vi "反控启动.vi"(10 "启动参数":T1(ring)=enum."CODCr", 11 "启动类型":T2(ring)) -> ()   [LabVIEW 2016]
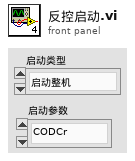
[diagram p1: front panel]
types:
  T1 = enum16{"未选择", "CODMn", "氨氮", "总磷", "总氮", "CODCr"}
  T2 = enum16{"启动整机", "停止整机", "标样核查", "加标回收", "平行样测试", "零点核查", "跨度核查", "校零", "校标"}
  T3 = cluster{"测量模式":enum16{"水样测量", "标样核查", "零点核查", "跨度核查", "空白测试", "加标回收", "平行样", "校零", "校标"}}
  T4 = cluster{"站号":u16, "量程切换":enum32{"H", "L", "AUTO"}, "控制命令":enum16{"启动测量", "标样核查", "零点核查", "跨度核查", "空白测试", "平行样测试", "加标回收", "空白校准", "标样校准", "初始化（清洗）", "停止测试", "仪器重启", "校时", "模式设置", "测量间隔设置"}, "模式设置":enum16{"待机", "连续模式", "周期模式", "定点模式", "受控模式", "手动模式"}, "测量间隔":u16}
  T5 = cluster{"status":bool, "代码":u16, "source":string}
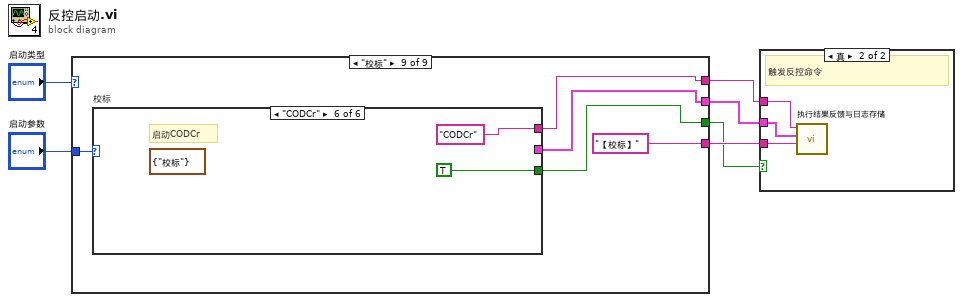
[diagram p0: block diagram]
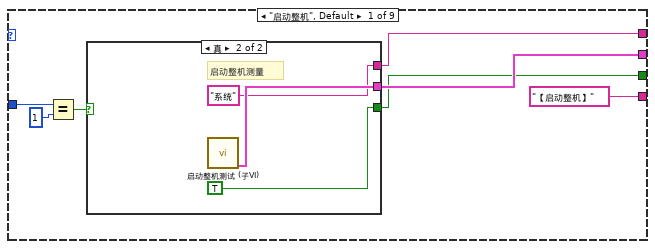
[diagram p3: hidden frame]
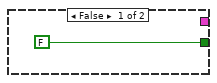
[diagram p4: hidden frame]
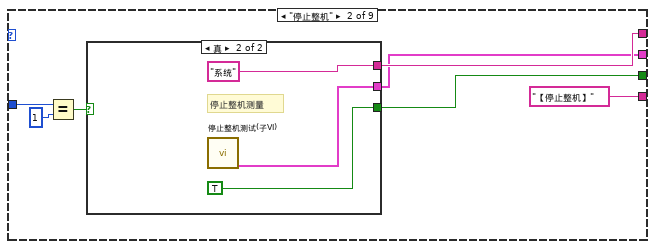
[diagram p5: hidden frame]
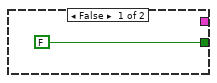
[diagram p6: hidden frame]
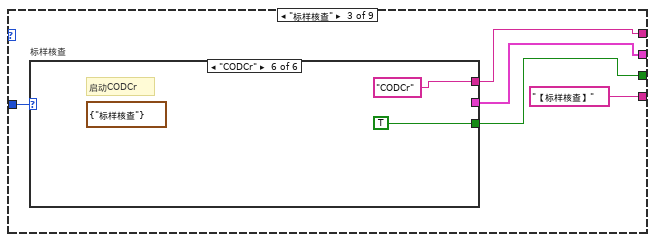
[diagram p7: hidden frame]
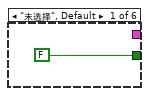
[diagram p8: hidden frame]
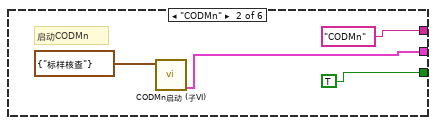
[diagram p9: hidden frame]
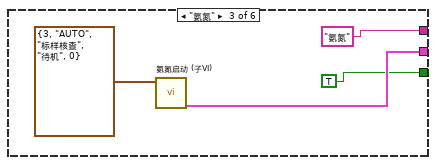
[diagram p10: hidden frame]
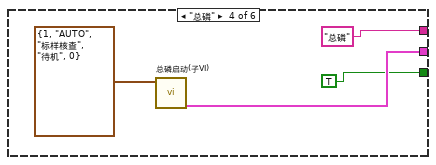
[diagram p11: hidden frame]
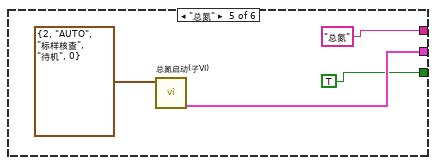
[diagram p12: hidden frame]
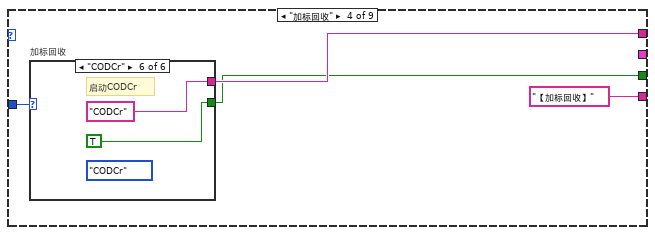
[diagram p13: hidden frame]
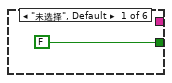
[diagram p14: hidden frame]
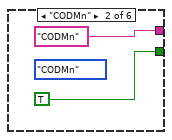
[diagram p15: hidden frame]
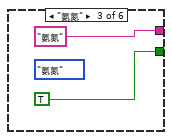
[diagram p16: hidden frame]
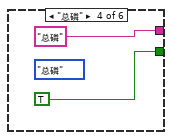
[diagram p17: hidden frame]
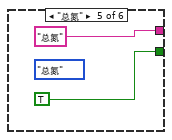
[diagram p18: hidden frame]
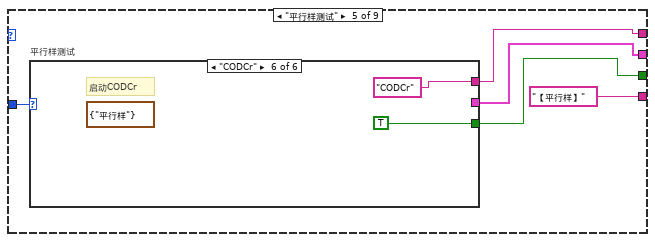
[diagram p19: hidden frame]
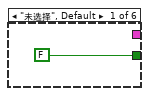
[diagram p20: hidden frame]
diagram:
  n1 = case shown="\"校标\"" "启动类型" {
    tunnel: "启动参数" -> [w13 w23 w33 w55 w72 w96 w120 w143 w168]
    tunnel: ["【启动整机】" ("日志信息") "【停止整机】" ("日志信息") "【标样核查】" ("日志信息") "【加标回收】" ("日志信息") "【平行样】" ("日志信息") "【零点核查】" ("日志信息") "【跨度核查】" ("日志信息") "【校零】" ("日志信息") "【校标】" ("日志信息")] -> w4
    tunnel: [w7 w19 w31 w53 w70 w93 w118 w141 w165] -> w3
    tunnel: [w10 w18 w30 _ w69 w94 w117 w140 w166] -> w2
    tunnel: [w8 w20 w32 w54 w68 w92 w119 w142 w164] -> w1
    frame "启动整机", Default {
      n2 = Equal?(x=w13, y=1) -> (x = y?=w11:bool)
      n3 = case shown="真" w11 {
        tunnel: [_ w17] -> w10
        tunnel: [_ "系统" ("设备")] -> w8
        tunnel: [FALSE TRUE] -> w7
        frame False {
        }
        frame True {
          # "启动整机测量"
          n4 = call "启动整机测试 (子VI).vi"() -> ("error out"=w17:T5)  [unwired: 11 in]
        }
      }
    }
    frame "停止整机" {
      n5 = Equal?(x=w23, y=1) -> (x = y?=w22:bool)
      n6 = case shown="真" w22 {
        tunnel: [_ "系统" ("设备")] -> w20
        tunnel: [FALSE TRUE] -> w19
        tunnel: [_ w26] -> w18
        frame False {
        }
        frame True {
          # "停止整机测量"
          n7 = call "停止整机测试(子VI).vi"() -> ("error out"=w26:T5)  [unwired: 11 in]
        }
      }
    }
    frame "标样核查" {
      n8 = case "标样核查" shown="\"CODCr\"" w33 {
        tunnel: [_ "CODMn" ("设备") "氨氮" ("设备") "总磷" ("设备") "总氮" ("设备") "CODCr" ("设备")] -> w32
        tunnel: [_ w37 w41 w44 w48 _] -> w30
        tunnel: [FALSE TRUE TRUE TRUE TRUE TRUE] -> w31
        frame "未选择", Default {
        }
        frame "CODMn" {
          # "启动CODMn"
          n9 = call "CODMn启动 (子VI).vi"("启动测量模式"=T3 {"测量模式"=enum."标样核查"}) -> ("error out"=w37:T5)  [unwired: 10 in]
        }
        frame "氨氮" {
          n10 = call "氨氮启动 (子VI).vi"("参数"=T4 {"站号"=3, "量程切换"=enum."AUTO", "控制命令"=enum."标样核查", "模式设置"=enum."待机", "测量间隔"=0}) -> ("error out"=w41:T5)  [unwired: 10 in]
        }
        frame "总磷" {
          n11 = call "总磷启动(子VI).vi"("参数"=T4 {"站号"=1, "量程切换"=enum."AUTO", "控制命令"=enum."标样核查", "模式设置"=enum."待机", "测量间隔"=0}) -> ("error out"=w44:T5)  [unwired: 10 in]
        }
        frame "总氮" {
          n12 = call "总氮启动(子VI).vi"("参数"=T4 {"站号"=2, "量程切换"=enum."AUTO", "控制命令"=enum."标样核查", "模式设置"=enum."待机", "测量间隔"=0}) -> ("error out"=w48:T5)  [unwired: 10 in]
        }
        frame "CODCr" {
          (unwired) T3 {"测量模式"=enum."标样核查"} ("启动测量模式")
          # "启动CODCr"
        }
      }
    }
    frame "加标回收" {
      n13 = case "加标回收" shown="\"CODCr\"" w55 {
        tunnel: [_ "CODMn" ("设备") "氨氮" ("设备") "总磷" ("设备") "总氮" ("设备") "CODCr" ("设备")] -> w54
        tunnel: [FALSE TRUE TRUE TRUE TRUE TRUE] -> w53
        frame "未选择", Default {
        }
        frame "CODMn" {
          (unwired) T1."CODMn" ("启动参数")
        }
        frame "氨氮" {
          (unwired) T1."氨氮" ("启动参数")
        }
        frame "总磷" {
          (unwired) T1."总磷" ("启动参数")
        }
        frame "总氮" {
          (unwired) T1."总氮" ("启动参数")
        }
        frame "CODCr" {
          (unwired) T1."CODCr" ("启动参数")
          # "启动CODCr"
        }
      }
    }
    frame "平行样测试" {
      n14 = case "平行样测试" shown="\"CODCr\"" w72 {
        tunnel: [_ "CODMn" ("设备") "氨氮" ("设备") "总磷" ("设备") "总氮" ("设备") "CODCr" ("设备")] -> w68
        tunnel: [_ w76 w80 w83 w87 _] -> w69
        tunnel: [FALSE TRUE TRUE TRUE TRUE TRUE] -> w70
        frame "未选择", Default {
        }
        frame "CODMn" {
          # "启动CODMn"
          n15 = call "CODMn启动 (子VI).vi"("启动测量模式"=T3 {"测量模式"=enum."平行样"}) -> ("error out"=w76:T5)  [unwired: 10 in]
        }
        frame "氨氮" {
          n16 = call "氨氮启动 (子VI).vi"("参数"=T4 {"站号"=3, "量程切换"=enum."AUTO", "控制命令"=enum."平行样测试", "模式设置"=enum."待机", "测量间隔"=0}) -> ("error out"=w80:T5)  [unwired: 10 in]
        }
        frame "总磷" {
          n17 = call "总磷启动(子VI).vi"("参数"=T4 {"站号"=1, "量程切换"=enum."AUTO", "控制命令"=enum."平行样测试", "模式设置"=enum."待机", "测量间隔"=0}) -> ("error out"=w83:T5)  [unwired: 10 in]
        }
        frame "总氮" {
          n18 = call "总氮启动(子VI).vi"("参数"=T4 {"站号"=2, "量程切换"=enum."AUTO", "控制命令"=enum."平行样测试", "模式设置"=enum."待机", "测量间隔"=0}) -> ("error out"=w87:T5)  [unwired: 10 in]
        }
        frame "CODCr" {
          (unwired) T3 {"测量模式"=enum."平行样"} ("启动测量模式")
          # "启动CODCr"
        }
      }
    }
    frame "零点核查" {
      n19 = case "零点核查" shown="\"CODCr\"" w96 {
        tunnel: [_ "CODMn" ("设备") "氨氮" ("设备") "总磷" ("设备") "总氮" ("设备") "CODCr" ("设备")] -> w92
        tunnel: [_ w100 w104 w107 w111 _] -> w94
        tunnel: [FALSE TRUE TRUE TRUE TRUE TRUE] -> w93
        frame "未选择", Default {
        }
        frame "CODMn" {
          # "启动CODMn"
          n20 = call "CODMn启动 (子VI).vi"("启动测量模式"=T3 {"测量模式"=enum."零点核查"}) -> ("error out"=w100:T5)  [unwired: 10 in]
        }
        frame "氨氮" {
          n21 = call "氨氮启动 (子VI).vi"("参数"=T4 {"站号"=3, "量程切换"=enum."AUTO", "控制命令"=enum."零点核查", "模式设置"=enum."待机", "测量间隔"=0}) -> ("error out"=w104:T5)  [unwired: 10 in]
        }
        frame "总磷" {
          n22 = call "总磷启动(子VI).vi"("参数"=T4 {"站号"=1, "量程切换"=enum."AUTO", "控制命令"=enum."零点核查", "模式设置"=enum."待机", "测量间隔"=0}) -> ("error out"=w107:T5)  [unwired: 10 in]
        }
        frame "总氮" {
          n23 = call "总氮启动(子VI).vi"("参数"=T4 {"站号"=2, "量程切换"=enum."AUTO", "控制命令"=enum."零点核查", "模式设置"=enum."待机", "测量间隔"=0}) -> ("error out"=w111:T5)  [unwired: 10 in]
        }
        frame "CODCr" {
          (unwired) T3 {"测量模式"=enum."零点核查"} ("启动测量模式")
          # "启动CODCr"
        }
      }
    }
    frame "跨度核查" {
      n24 = case "跨度核查" shown="\"CODCr\"" w120 {
        tunnel: [_ "CODMn" ("设备") "氨氮" ("设备") "总磷" ("设备") "总氮" ("设备") "CODCr" ("设备")] -> w119
        tunnel: [_ w124 w128 w131 w135 _] -> w117
        tunnel: [FALSE TRUE TRUE TRUE TRUE TRUE] -> w118
        frame "未选择", Default {
        }
        frame "CODMn" {
          # "启动CODMn"
          n25 = call "CODMn启动 (子VI).vi"("启动测量模式"=T3 {"测量模式"=enum."跨度核查"}) -> ("error out"=w124:T5)  [unwired: 10 in]
        }
        frame "氨氮" {
          n26 = call "氨氮启动 (子VI).vi"("参数"=T4 {"站号"=3, "量程切换"=enum."AUTO", "控制命令"=enum."跨度核查", "模式设置"=enum."待机", "测量间隔"=0}) -> ("error out"=w128:T5)  [unwired: 10 in]
        }
        frame "总磷" {
          n27 = call "总磷启动(子VI).vi"("参数"=T4 {"站号"=1, "量程切换"=enum."AUTO", "控制命令"=enum."跨度核查", "模式设置"=enum."待机", "测量间隔"=0}) -> ("error out"=w131:T5)  [unwired: 10 in]
        }
        frame "总氮" {
          n28 = call "总氮启动(子VI).vi"("参数"=T4 {"站号"=2, "量程切换"=enum."AUTO", "控制命令"=enum."跨度核查", "模式设置"=enum."待机", "测量间隔"=0}) -> ("error out"=w135:T5)  [unwired: 10 in]
        }
        frame "CODCr" {
          (unwired) T3 {"测量模式"=enum."跨度核查"} ("启动测量模式")
          # "启动CODCr"
        }
      }
    }
    frame "校零" {
      n29 = case "校零" shown="\"CODCr\"" w143 {
        tunnel: [_ "CODMn" ("设备") "氨氮" ("设备") "总磷" ("设备") "总氮" ("设备") "CODCr" ("设备")] -> w142
        tunnel: [_ w148 w152 w155 w159 _] -> w140
        tunnel: [FALSE TRUE TRUE TRUE TRUE TRUE] -> w141
        frame "未选择", Default {
        }
        frame "CODMn" {
          # "启动CODMn"
          n30 = call "CODMn启动 (子VI).vi"("启动测量模式"=T3 {"测量模式"=enum."校零"}) -> ("error out"=w148:T5)  [unwired: 10 in]
        }
        frame "氨氮" {
          n31 = call "氨氮启动 (子VI).vi"("参数"=T4 {"站号"=3, "量程切换"=enum."AUTO", "控制命令"=enum."空白校准", "模式设置"=enum."待机", "测量间隔"=0}) -> ("error out"=w152:T5)  [unwired: 10 in]
        }
        frame "总磷" {
          n32 = call "总磷启动(子VI).vi"("参数"=T4 {"站号"=1, "量程切换"=enum."AUTO", "控制命令"=enum."空白校准", "模式设置"=enum."待机", "测量间隔"=0}) -> ("error out"=w155:T5)  [unwired: 10 in]
        }
        frame "总氮" {
          n33 = call "总氮启动(子VI).vi"("参数"=T4 {"站号"=2, "量程切换"=enum."AUTO", "控制命令"=enum."空白校准", "模式设置"=enum."待机", "测量间隔"=0}) -> ("error out"=w159:T5)  [unwired: 10 in]
        }
        frame "CODCr" {
          (unwired) T3 {"测量模式"=enum."校零"} ("启动测量模式")
          # "启动CODCr"
        }
      }
    }
    frame "校标" {
      n34 = case "校标" shown="\"CODCr\"" w168 {
        tunnel: [_ "CODMn" ("设备") "氨氮" ("设备") "总磷" ("设备") "总氮" ("设备") "CODCr" ("设备")] -> w164
        tunnel: [_ w172 w176 w179 w183 _] -> w166
        tunnel: [FALSE TRUE TRUE TRUE TRUE TRUE] -> w165
        frame "未选择", Default {
        }
        frame "CODMn" {
          # "启动CODMn"
          n35 = call "CODMn启动 (子VI).vi"("启动测量模式"=T3 {"测量模式"=enum."校标"}) -> ("error out"=w172:T5)  [unwired: 10 in]
        }
        frame "氨氮" {
          n36 = call "氨氮启动 (子VI).vi"("参数"=T4 {"站号"=3, "量程切换"=enum."AUTO", "控制命令"=enum."标样校准", "模式设置"=enum."待机", "测量间隔"=0}) -> ("error out"=w176:T5)  [unwired: 10 in]
        }
        frame "总磷" {
          n37 = call "总磷启动(子VI).vi"("参数"=T4 {"站号"=1, "量程切换"=enum."AUTO", "控制命令"=enum."标样校准", "模式设置"=enum."待机", "测量间隔"=0}) -> ("error out"=w179:T5)  [unwired: 10 in]
        }
        frame "总氮" {
          n38 = call "总氮启动(子VI).vi"("参数"=T4 {"站号"=2, "量程切换"=enum."AUTO", "控制命令"=enum."标样校准", "模式设置"=enum."待机", "测量间隔"=0}) -> ("error out"=w183:T5)  [unwired: 10 in]
        }
        frame "CODCr" {
          (unwired) T3 {"测量模式"=enum."校标"} ("启动测量模式")
          # "启动CODCr"
        }
      }
    }
  }
  n39 = case shown="真" w3 {
    tunnel: w4 -> [_ w188]
    tunnel: w2 -> [_ w189]
    tunnel: w1 -> [_ w190]
    frame False {
    }
    frame True {
      # "触发反控命令"
      n40 = call "执行结果反馈与日志存储.vi"("日志信息"=w188, "error out"=w189, "设备"=w190) -> ()  [unwired: 9 in]
    }
  }
